vi "1-18.vi"() -> ()   [LabVIEW 2022 SP3]
panel:
  out "等于":dbl
  in  "数值 2":dbl
  in  "数值":dbl
  in  "下拉列表":u16(ring) items=["+", "-"]
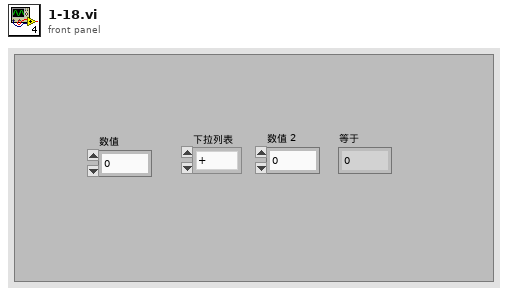
[diagram p1: front panel]
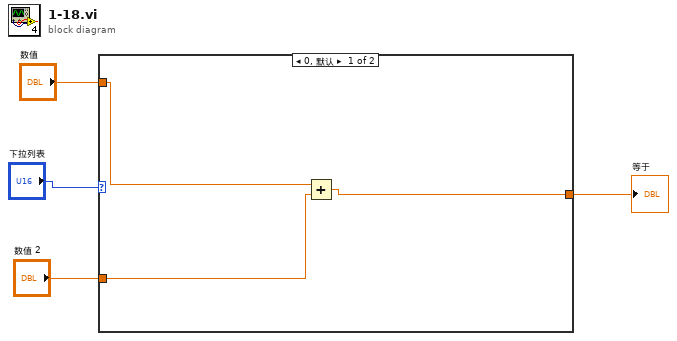
[diagram p0: block diagram]
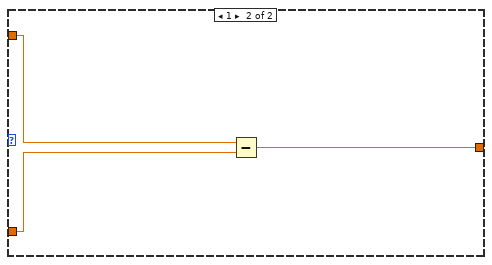
[diagram p2: hidden frame]
diagram:
  n1 = case "条件结构" shown="0, 默认" "下拉列表" {
    tunnel: "数值" -> [w7 w10]
    tunnel: "数值 2" -> [w6 w9]
    tunnel: [w5 w8] -> w1
    frame 0, Default {
      n2 = Add(x=w7, y=w6) -> (x+y=w5:dbl)
    }
    frame 1 {
      n3 = Subtract(x=w10, y=w9) -> (x-y=w8:dbl)
    }
  }
  "等于" <- w1
